vi "dfd_Nyquist Filter Design Make Response Positive.vi"(7 "#band":i32, 8 "error in (no error)":errorcluster, 11 "h in":dbl[](array[numeric])) -> (0 "error out":errorcluster, 3 "h out":dbl[](array[numeric]))   [LabVIEW 2017, in "NI_DigFilter_Process.lvlib"]
uses:
  <vilib>/addons/Digital Filter Design/NI_DigFilter_Process.lvlib
  <vilib>/addons/Digital Filter Design/NI_DigFilterLicensed.lvlib
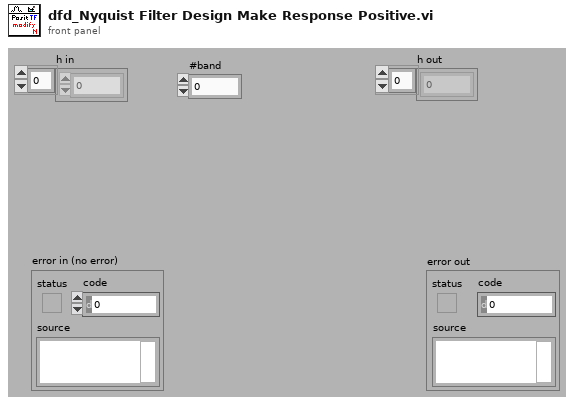
[diagram p1: front panel]
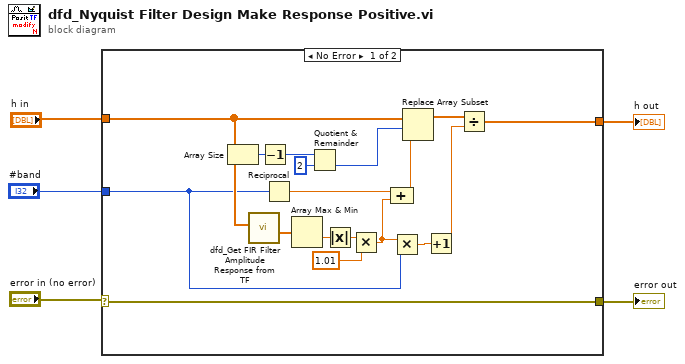
[diagram p0: block diagram]
diagram:
  n1 = case shown="No Error" "error in (no error)" {
    selector: "error in (no error)" -> [w9 w24]
    tunnel: "#band" -> [w6 _]
    tunnel: "h in" -> [w11 _]
    tunnel: [w10 _] -> w1
    tunnel: [w9 w24] -> w2
    frame No Error {
      n2 = Array Size(array=w11) -> (size(s)=w21:i32)
      n3 = call <vilib>:"dfd_Get FIR Filter Amplitude Response from TF.vi"("numerator"=w11) -> ("Amplitude"=w15:dbl[])  [unwired: 1 in, 9 out]
      n4 = Decrement(x=w21) -> (x-1=w17:i32)
      n5 = Reciprocal(x=w6) -> (1/x=w16:dbl)
      n6 = Array Max & Min(array=w15) -> (min value=w14:dbl)  [unwired: 3 out]
      n7 = Quotient & Remainder(x=w17, y=2) -> (floor(x/y)=w20:i32)  [unwired: 1 out]
      n8 = Absolute Value(x=w14) -> (abs(x)=w13:dbl)
      n9 = Multiply(x=w13, y=1.01) -> (x*y=w7:dbl)
      n10 = Compound Arithmetic op=ADD(w16, w7) -> (w23:dbl)
      n11 = Multiply(x=w7, y=w6) -> (x*y=w8:dbl)
      n12 = Replace Array Subset(array=w11, new element=w23, index=w20) -> (w18:dbl[])
      n13 = Increment(x=w8) -> (x+1=w19:dbl)
      n14 = Divide(x=w18, y=w19) -> (x/y=w10:dbl[])
    }
    frame Error {
    }
  }
  "error out" <- w2
  "h out" <- w1
